vi "WLAN - TV - OPPO - RW - ReadTestVectorFile(Rx).vi"(5 "Rx Measurements Settings":T2 {"DSSS Data Rate (Mbps)" items=["1", "2", "5.5 CCK", "5.5 PBCC", "11 CCK", "11 PBCC", "22", "33"]; "OFDM Data Rate (Mbps)" items=["6", "9", "12", "18", "24", "36", "48", "54"]; "80211n PLCP Frame Format" items=["Mixed Format", "Greenfield Format"]}) -> (8 "Waveform Generation Settings":T1 {"DSSS Data Rate (Mbps)" items=["1", "2", "5.5 CCK", "5.5 PBCC", "11 CCK", "11 PBCC", "22", "33"]; "OFDM Data Rate (Mbps)" items=["6", "9", "12", "18", "24", "36", "48", "54"]; "80211n PLCP Frame Format" items=["Mixed Format", "Greenfield Format"]; "Standard" items=["80211A/G/J/P OFDM", "80211B/G DSSS", "80211G DSSSOFDM", "80211N MIMOOFDM", "80211AC MIMOOFDM"]})   [LabVIEW 2012]
uses:
  Includes/WLAN - TV - OPPO - RW - INC - TV_Rx_Measurements.ctl
  Includes/WLAN - NIStandardDefine.ctl
  Includes/WLAN - TV - RW - INC - Rx_PER_Wfm_Settings.ctl
panel:
  in  "Wfm_Index":i32
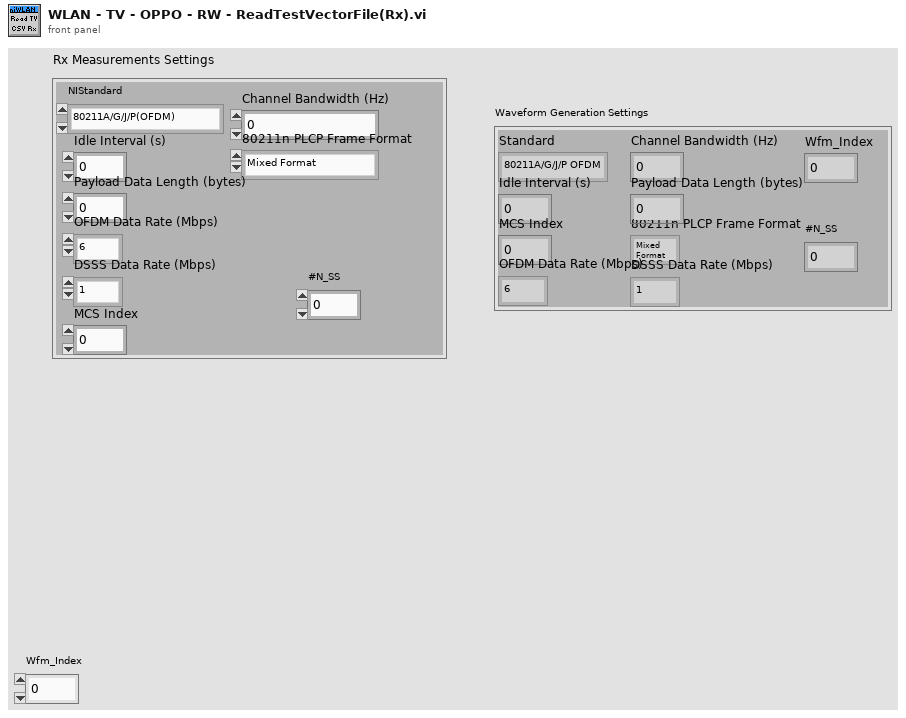
[diagram p1: front panel]
types:
  T1 = typedef "WLAN - TV - RW - INC - Rx_PER_Wfm_Settings.ctl" = cluster{"Standard":i32, "Channel Bandwidth (Hz)":dbl, "Idle Interval (s)":dbl, "MCS Index":i32, "80211n PLCP Frame Format":i32, "Payload Data Length (bytes)":i32, "OFDM Data Rate (Mbps)":i32, "DSSS Data Rate (Mbps)":i32, "Wfm_Index":i32, "#N_SS":i32}
  T2 = typedef "WLAN - TV - OPPO - RW - INC - TV_Rx_Measurements.ctl" = cluster{"Channel Bandwidth (Hz)":dbl, "Idle Interval (s)":dbl, "MCS Index":i32, "80211n PLCP Frame Format":i32, "Payload Data Length (bytes)":i32, "OFDM Data Rate (Mbps)":i32, "DSSS Data Rate (Mbps)":i32, "#N_SS":i32, "NIStandard":T3}
  T3 = typedef "WLAN - NIStandardDefine.ctl" = enum32{"80211A/G/J/P(OFDM)", "80211B/G(DSSS)", "80211GDSSSOFDM", "80211NMIMOOFDM", "80211ACMIMOOFDM"}
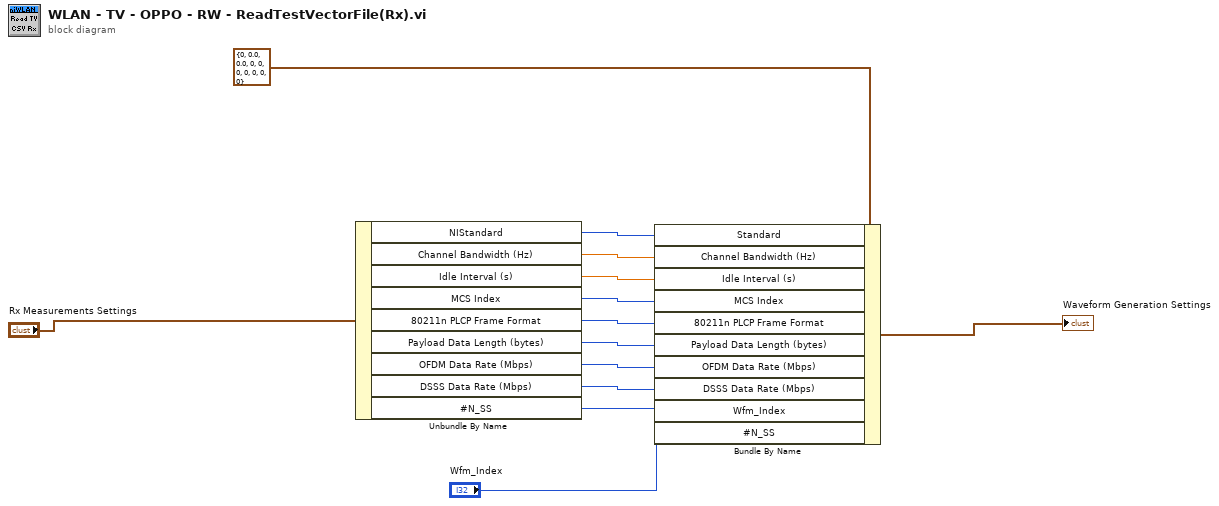
[diagram p0: block diagram]
diagram:
  n1 = Unbundle By Name("Rx Measurements Settings") -> ("NIStandard"=w11:T3, "Channel Bandwidth (Hz)"=w10:dbl, "Idle Interval (s)"=w9:dbl, "MCS Index"=w4:i32, "80211n PLCP Frame Format"=w5:i32, "Payload Data Length (bytes)"=w6:i32, "OFDM Data Rate (Mbps)"=w7:i32, "DSSS Data Rate (Mbps)"=w8:i32, "#N_SS"=w1:i32)
  n2 = Bundle By Name(cluster=T1 {"Standard"=0, "Channel Bandwidth (Hz)"=0.0, "Idle Interval (s)"=0.0, "MCS Index"=0, "80211n PLCP Frame Format"=0, "Payload Data Length (bytes)"=0, "OFDM Data Rate (Mbps)"=0, "DSSS Data Rate (Mbps)"=0, "Wfm_Index"=0, "#N_SS"=0} ("Rx Measurements Settings"), "Standard"=w11, "Channel Bandwidth (Hz)"=w10, "Idle Interval (s)"=w9, "MCS Index"=w4, "80211n PLCP Frame Format"=w5, "Payload Data Length (bytes)"=w6, "OFDM Data Rate (Mbps)"=w7, "DSSS Data Rate (Mbps)"=w8, "Wfm_Index"="Wfm_Index", "#N_SS"=w1) -> (→"Waveform Generation Settings":T1)
